vi "Test Parse 2xSpace Delimited Array.vi"(8 "error in (no error)":errorcluster, 11 "Test Case In":refnum<class "Helpers Test.lvclass">) -> (0 "error out":errorcluster, 3 "Test Case Out":refnum<class "Helpers Test.lvclass">)   [LabVIEW 2020, in "Helpers Test.lvclass"]
uses:
  Helpers Test.lvclass
  4993e8ee-a06a-463a-9684-69129f64d5ce.vi
  Helpers.lvlib
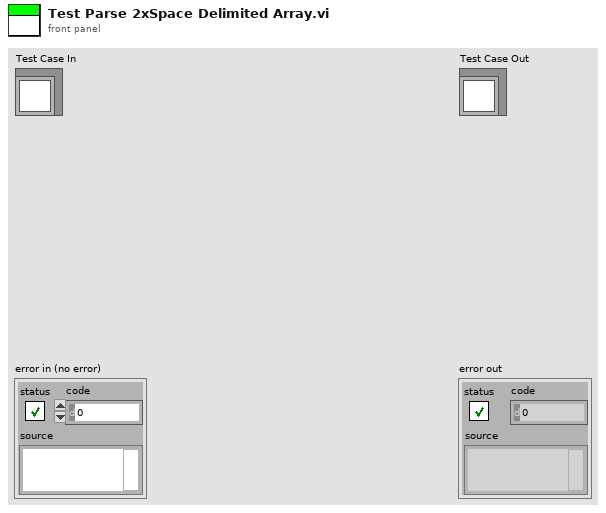
[diagram p1: front panel]
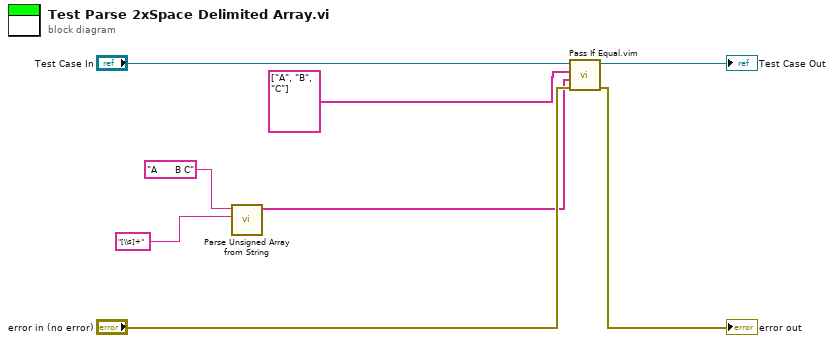
[diagram p0: block diagram]
diagram:
  n1 = call "Parse Unsigned Array from String.vi"("Delimiter regex"="[\\s]+", "Input"="A      B C") -> ("Parsed Array"=w3:string[])  [unwired: 8 in, 1 out]
  n2 = call "Pass If Equal.vim"("error in (no error)"="error in (no error)", "Actual"=w3, "Expected"=string[] ["A", "B", "C"] ("Parsed Array"), "LUnit Test Case In"="Test Case In") -> ("error out"=→"error out":errorcluster, "LUnit Test Case Out"=→"Test Case Out":refnum<class "Helpers Test.lvclass">)  [unwired: 6 in]
